vi "Close by Reference.vi"(8 "error in (no error)":errorcluster, 11 "CIPC Reference":u64) -> (0 "error out":errorcluster)   [LabVIEW 2021, in "CIF_NI_CIPC.lvlib"]
doc: "Close the reference to the buffer without destroying the buffer."
uses:
  CIF_NI_CIPC.lvlib
  <vilib>/Utility/error.llb/Trim Whitespace.vi
  <vilib>/Utility/error.llb/Error Cluster From Error Code.vi
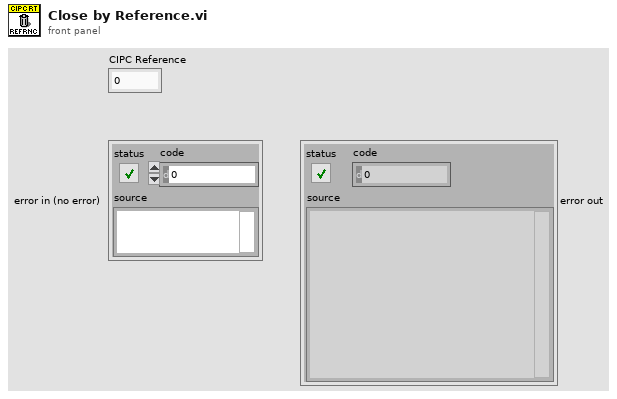
[diagram p1: front panel]
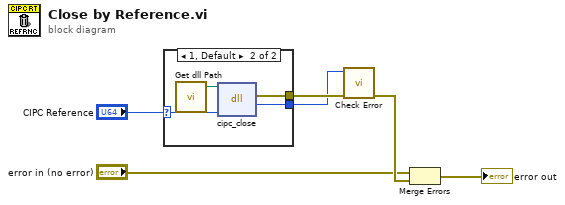
[diagram p0: block diagram]
diagram:
  n1 = case shown="1, Default" "CIPC Reference" {
    selector: "CIPC Reference" -> [_ w8]
    tunnel: [_ w10] -> w6
    tunnel: [_ w9] -> w5
    frame 0 {
    }
    frame 1, Default {
      n2 = call "Get dll Path.vi"() -> ("appended path"=w7:path)  [unwired: 5 in]
      n3 = dll-call lib="libnicipc.*" fn="cipc_close"(path in=w7, "cipc_buffer_ref"=w8) -> (error out=w10:errorcluster, "return type"=w9:i32)  [unwired: 3 in, 1 out]
    }
  }
  n4 = call "Check Error.vi"("error in (no error)"=w6, "Error Code"=w5) -> ("error out"=w4:errorcluster)  [unwired: 9 in]
  n5 = Merge Errors("error in (no error)", w4) -> (→"error out":errorcluster)
